vi "fluxo_dados.vi"() -> ()   [LabVIEW 2013]
panel:
  out "x-y":dbl
  in  "y":dbl
  in  "x":dbl
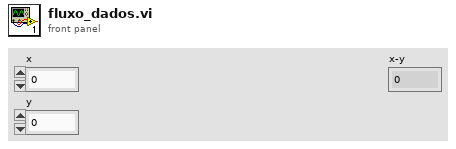
[diagram p1: front panel]
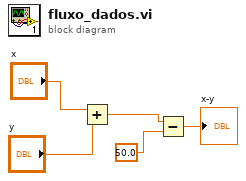
[diagram p0: block diagram]
diagram:
  n1 = Add(x="x", y="y") -> (x+y=w4:dbl)
  n2 = Subtract(x=w4, y=50.0) -> (x-y=→"x-y":dbl)
